vi "Read Pointer.vi"(8 "error in (no error)":errorcluster, 11 "Source in":refnum<class "Source.lvclass">) -> (0 "error out":errorcluster, 2 "source pointer":i64, 3 "Source out":refnum<class "Source.lvclass">)   [LabVIEW 2020, in "Server.lvlib" / "Source.lvclass"]
uses:
  Source.lvclass
  Source.lvclass/Source.ctl
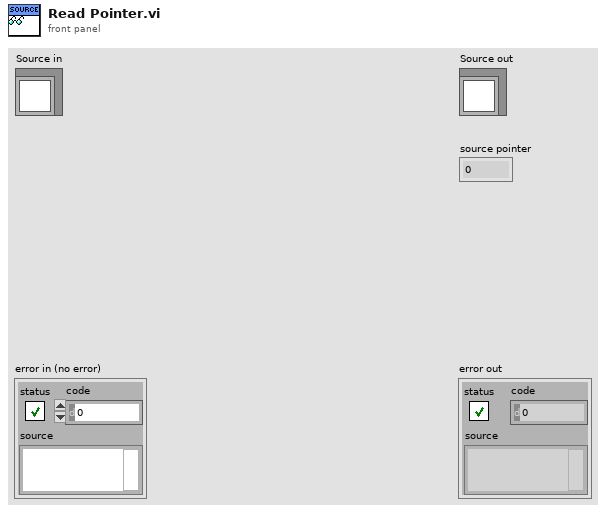
[diagram p1: front panel]
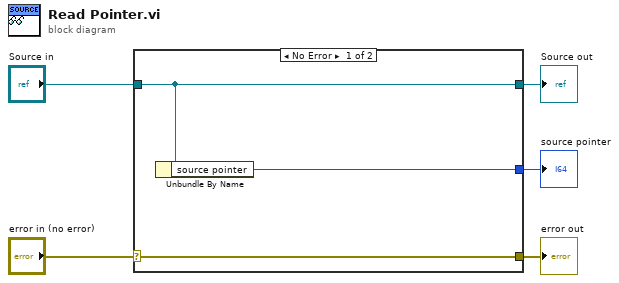
[diagram p0: block diagram]
diagram:
  n1 = case shown="No Error" "error in (no error)" {
    selector: "error in (no error)" -> [w8 w9]
    tunnel: [w8 w9] -> w4
    tunnel: [w7 w10] -> w2
    tunnel: "Source in" -> [w7 w10]
    tunnel: [w6 _] -> w1
    frame No Error {
      n2 = Unbundle By Name(w7) -> ("source pointer"=w6:i64)
    }
    frame Error {
    }
  }
  "error out" <- w4
  "Source out" <- w2
  "source pointer" <- w1
